vi "measure_element.vi"(8 "error in (no error)":errorcluster caption="エラー入力（エラーなし）", 9 "コマンド":string, 10 "文字送り間隔 (200 ms)":i16=200, 11 "VISAリソース名":refnum<visa-resource-name>) -> (0 "error out":errorcluster caption="エラー出力", 2 "読み取り":string, 3 "VISAリソース名 （出力）":refnum<visa-resource-name>)   [LabVIEW 2017]
panel:
  out "数値":i16
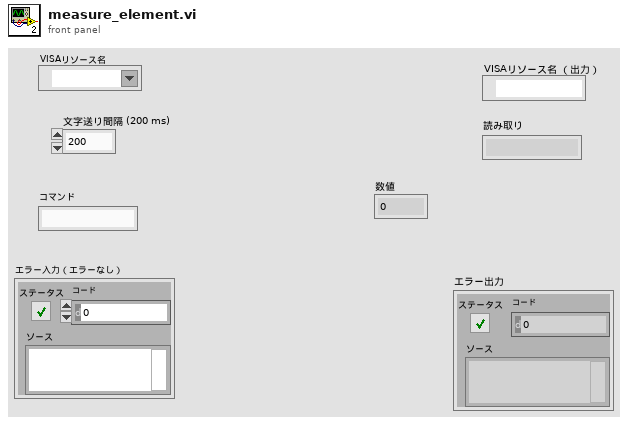
[diagram p1: front panel]
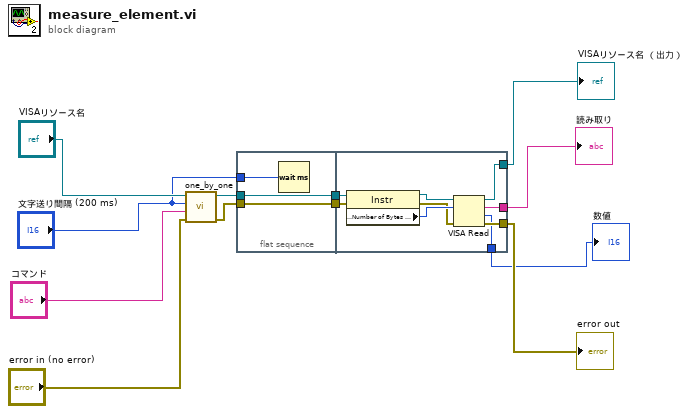
[diagram p0: block diagram]
diagram:
  n1 = call "one_by_one.vi"("error in (no error)"="error in (no error)", "入力文字"="コマンド", "待機 (200ms)"="文字送り間隔 (200 ms)", "VISAリソース名"="VISAリソース名") -> ("error out"=w11:errorcluster, "VISAリソース名出力"=w12:refnum<visa-resource-name>)  [unwired: 6 in]
  n2 = flat-sequence {
    tunnel: w11 -> [w14]
    tunnel: w12 -> [w15]
    tunnel: [w15] -> w5
    tunnel: [w14] -> w4
    tunnel: "文字送り間隔 (200 ms)" -> [w13]
    tunnel: [w19] -> w7
    tunnel: [w18] -> w6
    tunnel: w5 -> [w24]
    tunnel: w4 -> [w23]
    tunnel: [w17] -> w2
    tunnel: [w16] -> w1
    frame #0 {
      n3 = Wait (ms)(milliseconds to wait=w13) -> ()  [unwired: 1 out]
    }
    frame #1 {
      n4 = property class="Instr"(reference=w24, error in=w23) -> (reference out=w22:refnum<visa-resource-name>, error out=w20:errorcluster, "Serial Settings:Number of Bytes at Serial Port"=w21:u32)
      n5 = VISA Read(VISA resource name=w22, byte count=w21, error in (no error)=w20) -> (VISA resource name out=w19:refnum<visa-resource-name>, read buffer=w18:string, return count=w16:u32, error out=w17:errorcluster)
    }
  }
  "読み取り" <- w6
  "VISAリソース名 （出力）" <- w7
  "error out" <- w2
  "数値" <- w1
